vi "Begin.vi"(8 "error in":errorcluster) -> (0 "error out":errorcluster)   [LabVIEW 2017]
doc: "Called before other user functions, this VI is expected to open initial I/O refnums, load in file data, and do all program initialization. Notice that the <B>error out</B> terminal is simply used for data flow. Wiring it to other structures or subVIs ensures that this VI runs first."
uses:
  <vilib>/Rock Robotics/WPI/DriverStation/WPI_DriverStationRobotMode2.ctl
  Motor Enums.ctl
  <vilib>/Rock Robotics/SystemInterfaces/DIO/FPGA_DIOPWMChannel.ctl
  <vilib>/Rock Robotics/WPI/Joystick/WPI_JoystickDeviceEnum.ctl
  Robot Global Data.vi
  <vilib>/Rock Robotics/WPI/MotorControl/WPI_MotorControlOpen VictorSP.vi
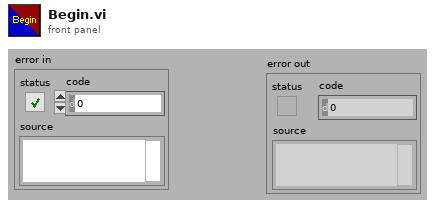
[diagram p1: front panel]
types:
  T1 = typedef "Motor Enums.ctl" = enum16{"drive joystick", "arm joystick", "left motor", "right motor", "elevator", "lever", "claw"}
  T2 = typedef "WPI_JoystickDeviceEnum.ctl" = enum16{"USB 0", "USB 1", "USB 2", "USB 3", "USB 4", "USB 5"}
  T3 = typedef "FPGA_DIOPWMChannel.ctl" = enum8{"PWM 0", "PWM 1", "PWM 2", "PWM 3", "PWM 4", "PWM 5", "PWM 6", "PWM 7", "PWM 8", "PWM 9", "PWM MXP 0", "PWM MXP 1", "PWM MXP 2", "PWM MXP 3", "PWM MXP 4", "PWM MXP 5", "PWM MXP 6", "PWM MXP 7", "PWM MXP 8", "PWM MXP 9", "Invalid"}
  T4 = typedef "WPI_DriverStationRobotMode2.ctl" = enum16{"Autonomous Disabled", "Autonomous Enabled", "Teleop Disabled", "Teleop Enabled", "Disconnected", "Finish", "Test Disabled", "Test Enabled", "Emergency Stopped"}
  T5 = typedef "WPI_MotorControlDeviceRef.ctl" = cluster{"DeviceStatus":errorcluster, "Type":T6, "PWM":cluster{"PWM Channel":T3, "DeadBand":T7}, "CAN":cluster{"Device Number":u8, "SetOutput VI Ref":variant, "GetOutput VI Ref":variant, "Enable VI Ref":variant, "Disable VI Ref":variant, "Data":variant}, "Invert":bool, "DIO PWM":cluster{"PWM \"Enable\" Channel":T3, "DIOChannel":T8, "PWM Rate":dbl}}
  T6 = typedef "WPI_MotorControlType.ctl" = enum16{"PWM", "CAN", "DIO PWM"}
  T7 = typedef "WPI_PWMDeadband.ctl" = cluster{"Name":string, "maxPositivePwm":i32, "minPositivePwm":i32, "centerPwm":i32, "maxNegativePwm":i32, "minNegativePwm":i32, "angularRange":u16}
  T8 = typedef "FPGA_DIOChannel.ctl" = enum8{"DIO 0", "DIO 1", "DIO 2", "DIO 3", "DIO 4", "DIO 5", "DIO 6", "DIO 7", "DIO 8", "DIO 9", "DIO MXP 0", "DIO MXP 1", "DIO MXP 2", "DIO MXP 3", "DIO MXP 4", "DIO MXP 5", "DIO MXP 6", "DIO MXP 7", "DIO MXP 8", "DIO MXP 9", "DIO MXP 10", "DIO MXP 11", "DIO MXP 12", "DIO MXP 13", "DIO MXP 14", "DIO MXP 15", "SPI Port CS1", "SPI Port CS2", "SPI Port CS3", "SPI Port MISO", "SPI Port MOSI", "Invalid"}
  T9 = typedef "WPI_JoystickDevRef.ctl" = cluster{"Device":T2}
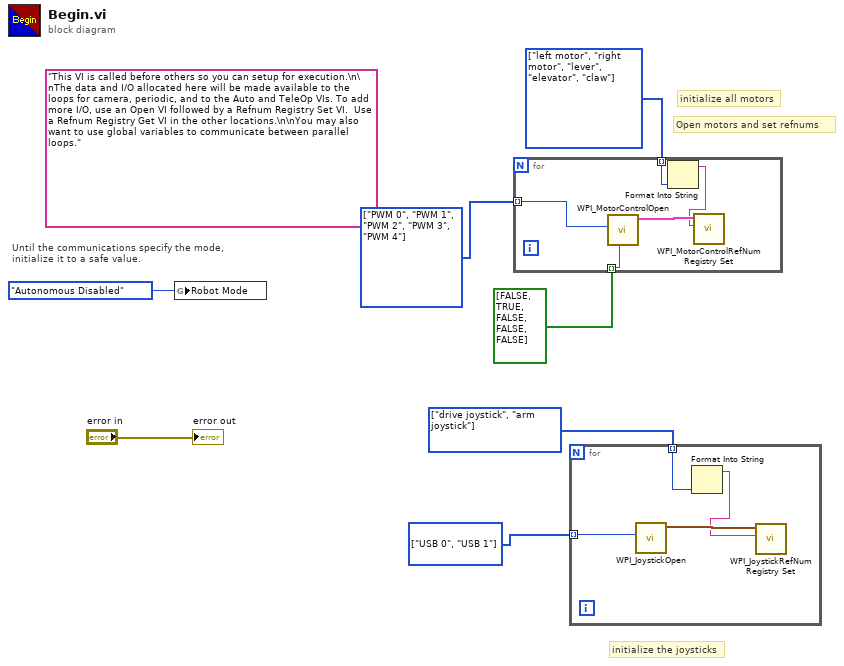
[diagram p0: block diagram]
diagram:
  w2 = T1[] [enum."drive joystick", enum."arm joystick"] items=["drive joystick", "arm joystick", "left motor", "right motor", "elevator", "lever", "claw"]
  w3 = T2[] [enum."USB 0", enum."USB 1"] items=["USB 0", "USB 1", "USB 2", "USB 3", "USB 4", "USB 5"] ("Array")
  w5 = T3[] [enum."PWM 0", enum."PWM 1", enum."PWM 2", enum."PWM 3", enum."PWM 4"] items=["PWM 0", "PWM 1", "PWM 2", "PWM 3", "PWM 4", "PWM 5", "PWM 6", "PWM 7", "PWM 8", "PWM 9", "PWM MXP 0", "PWM MXP 1", "PWM MXP 2", "PWM MXP 3", "PWM MXP 4", "PWM MXP 5", "PWM MXP 6", "PWM MXP 7", "PWM MXP 8", "PWM MXP 9", "Invalid"]
  w1 = T1[] [enum."left motor", enum."right motor", enum."lever", enum."elevator", enum."claw"] items=["drive joystick", "arm joystick", "left motor", "right motor", "elevator", "lever", "claw"]
  (unwired) "This VI is called before others so you can setup for execution.\n\nThe data and I/O allocated here will be made available to the loops for camera, periodic, and to the Auto and TeleOp VIs. To add more I/O, use an Open VI followed by a Refnum Registry Set VI.  Use a Refnum Registry Get VI in the other locations.\n\nYou may also want to use global variables to communicate between parallel loops."
  # "Open motors and set refnums"
  # "initialize the joysticks"
  # "Until the communications specify the mode,\ninitialize it to a safe value."
  # "initialize all motors"
  n1 = global write "Robot Global Data.vi" "Robot Mode"(WPI_DriverStationRobotMode2."Autonomous Disabled" ("Robot Mode")) -> ()
  n2 = for {
    tunnel: w5 -> [w12] mode=indexing
    tunnel: bool[] [FALSE, TRUE, FALSE, FALSE, FALSE] -> [w10] mode=indexing
    tunnel: w1 -> [w9] mode=indexing
    n3 = call-poly <vilib>:"WPI_MotorControlOpen.vi"("Invert"=w10, "PWM Channel"=w12) -> ("MotorControlDeviceRef"=w11:T5)  [unwired: 8 in, 1 out]
    n4 = Format Into String(w9) -> (resulting string=w8:string)  [unwired: 3 in, 1 out]
    n5 = call <vilib>:"WPI_MotorControlRefNum Registry Set.vi"("refnum name"=w8, "MotorControlDevRef"=w11) -> ()  [unwired: 8 in, 2 out]
  }
  n6 = for {
    tunnel: w3 -> [w15] mode=indexing
    tunnel: w2 -> [w14] mode=indexing
    n7 = call <vilib>:"WPI_JoystickOpen.vi"("JoystickDevice"=w15) -> ("JoystickDevRef"=w16:T9)  [unwired: 10 in]
    n8 = Format Into String(w14) -> (resulting string=w13:string)  [unwired: 3 in, 1 out]
    n9 = call <vilib>:"WPI_JoystickRefNum Registry Set.vi"("refnum name"=w13, "JoystickDevRef"=w16) -> ()  [unwired: 8 in, 2 out]
  }
  "error out" <- "error in"
